vi "uService GUI.vi"(8 "error in (no error)":errorcluster, 11 "uService Template in":refnum<class "Scheduler.lvclass">=refnum) -> (3 "uService Template out":refnum<class "Scheduler.lvclass">)   [LabVIEW 2020, in "CIRCUS_uServices.lvlib" / "Scheduler.lvlib" / "Scheduler.lvclass"]
uses:
  Scheduler.lvclass
  Scheduler Consumer Case Selector.ctl
  Selection.ctl
  TALOS/TALOS_PPL.lvlibp/Father of all uServices/Father of all uServices/Father of all uServices.lvclass
  C:/Users/marco/Documents/GitHub_Lab/CIRCUS/TALOS/TALOS_PPL.lvlibp/Father of all uServices/Father of all uServices/Father of all uServices.lvclass
  C:/Users/marco/Documents/GitHub_Lab/CIRCUS/TALOS/TALOS_PPL.lvlibp/Ancestor/Ancestor/Ancestor.lvclass
  C:/Users/marco/Documents/GitHub_Lab/CIRCUS/TALOS/Actor Framework.lvlibp/1abvi3w/vi.lib/ActorFramework/Actor/Actor.lvclass
  Run Utilities/Sequence of SBlocks/Sequence of SBlcoks - GUI.ctl
  Run Utilities/Sequence of SBlocks/Sequence of SBlocks.lvclass
  Run Utilities/TypeDefs/Synchronize FPGA Cluster.ctl
  Run Utilities/Run Utilities.lvlib
  Run Utilities/Schedule Block/Schedule Block - simplified GUI.ctl
  Run Utilities/Schedule Block/Schedule Block.lvclass
panel:
  out "Sync. mask":T1[](array[typedef])
  in  "SB Buttons":T2
  in  "Reload parameters":bool
  in  "Append to":enum32{"Bottom", "Top"}(radio)
  in  "Parallel":bool
  in  "Array of Sequences":T3[](array[typedef])
  in  "Science":bool
  in  "Save":bool
  in  "Load":bool
  in  "Reset":bool
  in  "Add RUN":bool
  in  "stop Scheduler":bool
  # "SCHEDULER"
  # "Multi FPGA Operation"
  # "Sync. mask"
  # "Estimated time of execution"
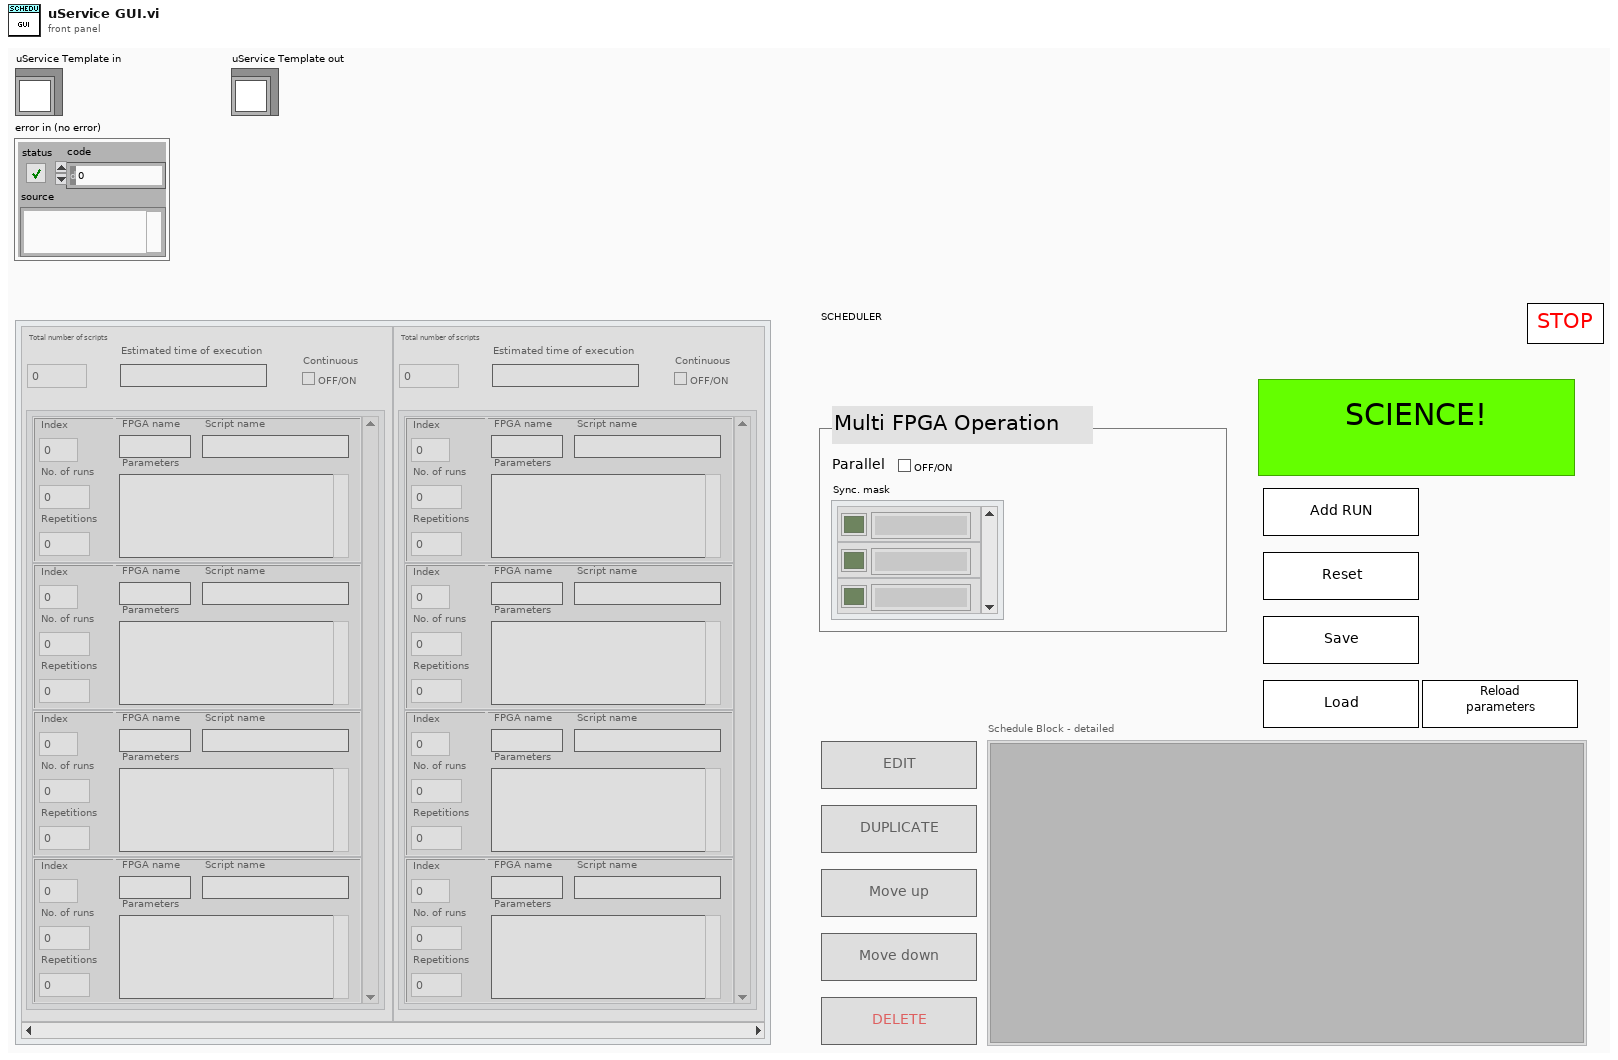
[diagram p1: front panel]
types:
  T1 = typedef "CIRCUS_uServices.lvlib/Run Utilities.lvlib/Synchronize FPGA Cluster.ctl" = cluster{"Status":bool, "FPGA Name":string}
  T2 = cluster{"Move up SB":bool, "Move down SB":bool, "DELETE_SB":bool, "DUPLICATE_SB":bool, "EDIT_SB":bool}
  T3 = typedef "CIRCUS_uServices.lvlib/Run Utilities.lvlib/Sequence of SBlocks.lvclass/Sequence of SBlcoks - GUI.ctl" = cluster{"Total number of scripts":i32, "Time":string, "Sequence of SBlocks":T4[], "Continuous":bool}
  T4 = typedef "CIRCUS_uServices.lvlib/Run Utilities.lvlib/Schedule Block.lvclass/Schedule Block - simplified GUI.ctl" = cluster{"Bcg Color":u32, "Index":i32, "No. of runs":i32, "Script name":string, "FPGA name":string, "Parameters":string, "Repetitions":i32}
  T5 = typedef "CIRCUS_uServices.lvlib/Scheduler.lvlib/Scheduler.lvclass/Scheduler Consumer Case Selector.ctl" = enum16{"Add SBlock", "Update GUI", "Move SBlock", "Select SBlock", "Update Cont.", "Load", "Save", "Reset", "Send to Tamer", "Edit SBlock", "Duplicate SBlock", "Delete SBlock", "Update SBlock", "Init", "Split/Combine Schedules", "Reschedule", "Load Parameters"}
  T6 = typedef "CIRCUS_uServices.lvlib/Scheduler.lvlib/Scheduler.lvclass/Selection.ctl" = cluster{"Row":i32, "Column":i32}
  T7 = typedef "TALOS.lvlib/Run Utilities.lvlib/Synchronize Kasli Cluster.ctl" = cluster{"Status":bool, "FPGA Name":string}
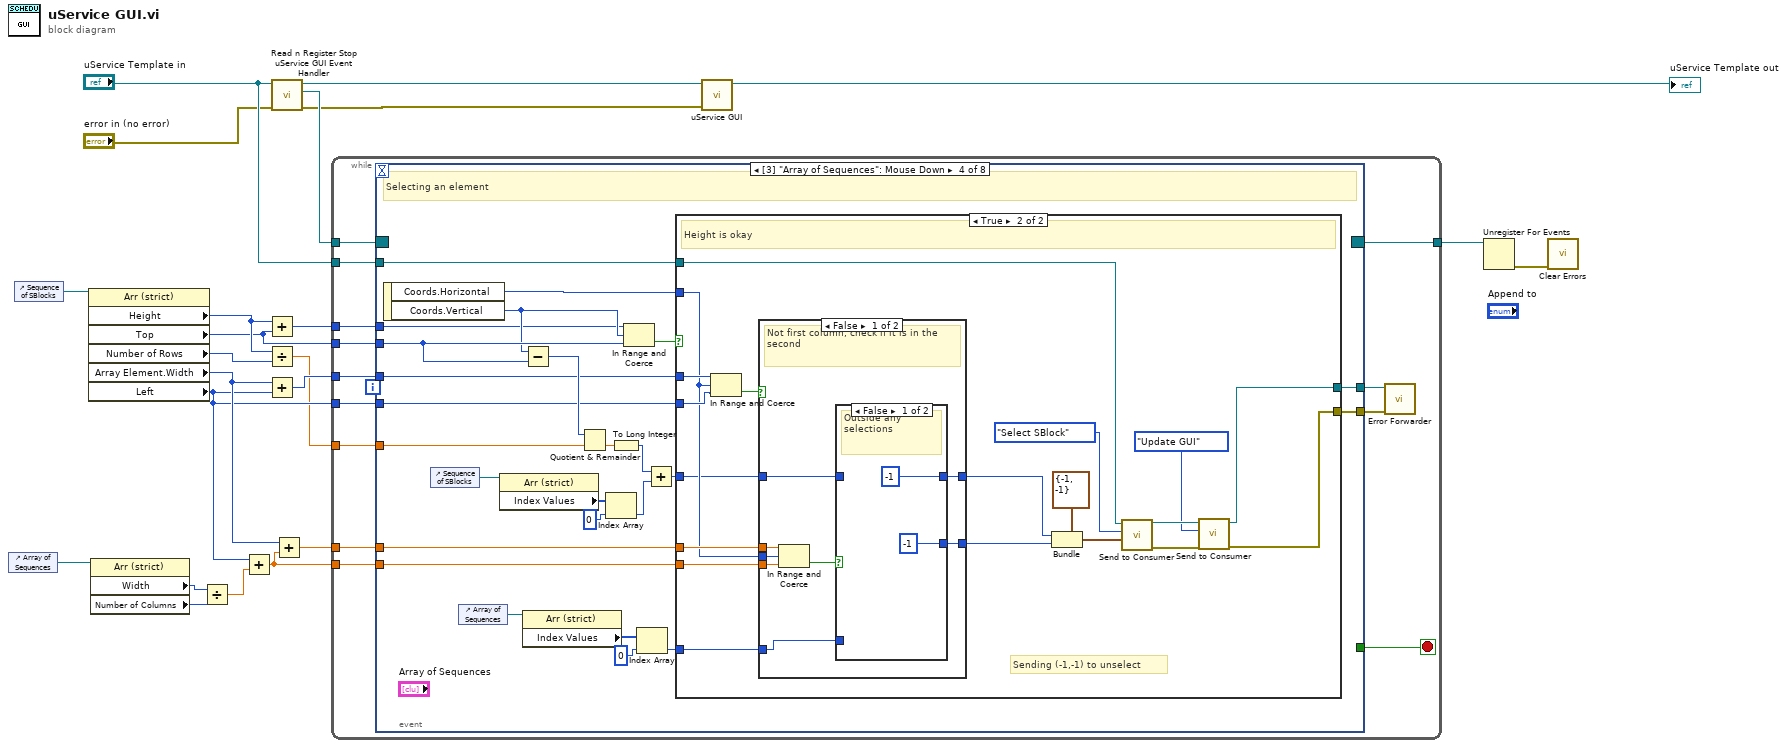
[diagram p0: block diagram]
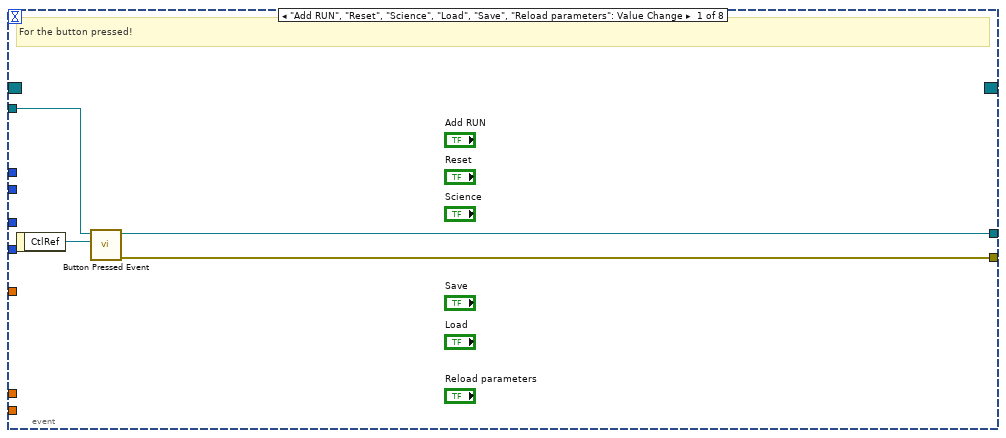
[diagram p2: hidden frame]
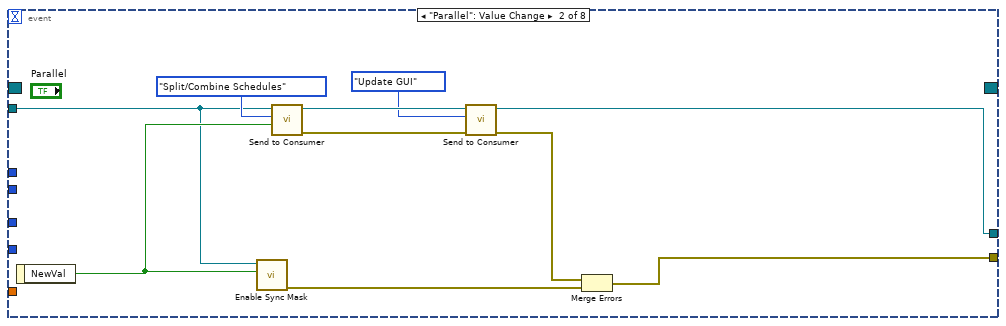
[diagram p3: hidden frame]
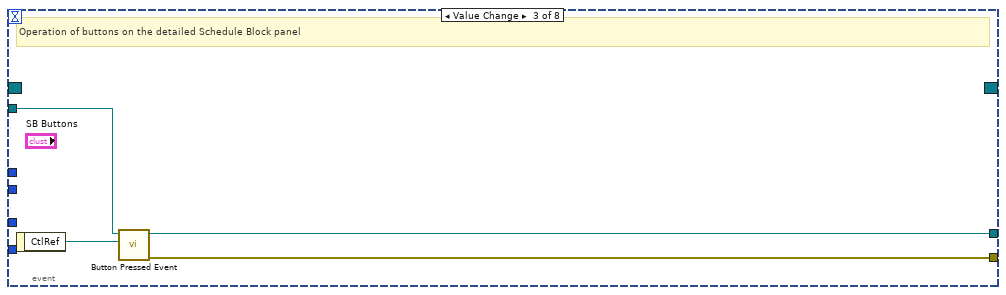
[diagram p4: hidden frame]
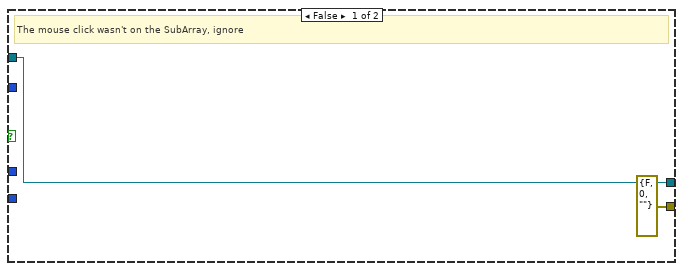
[diagram p5: hidden frame]
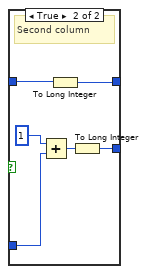
[diagram p6: hidden frame]
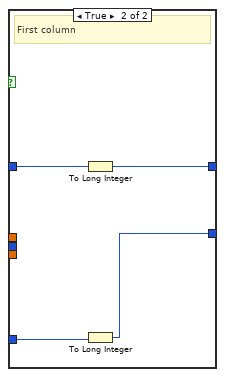
[diagram p7: hidden frame]
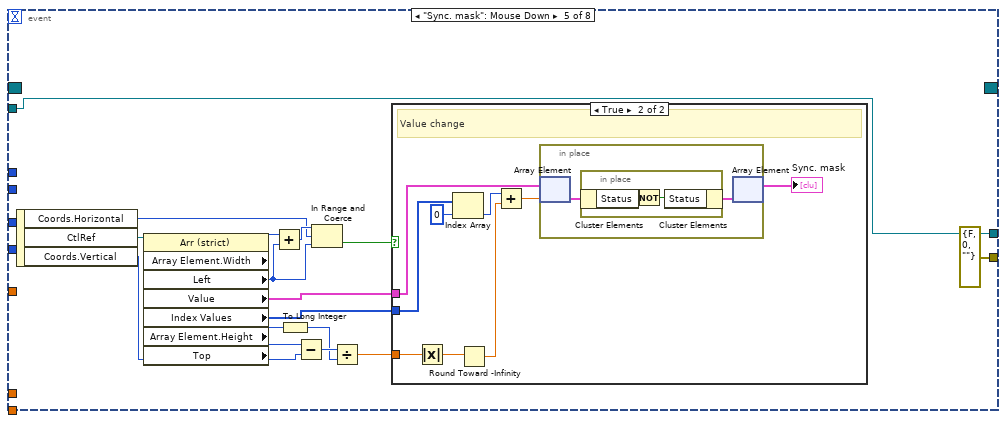
[diagram p8: hidden frame]
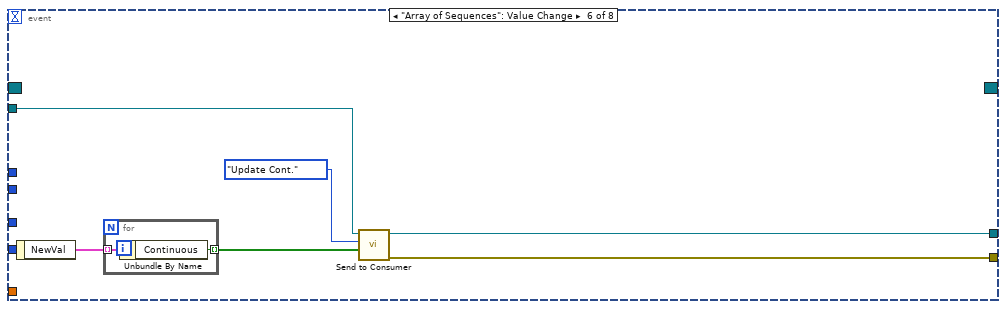
[diagram p10: hidden frame]
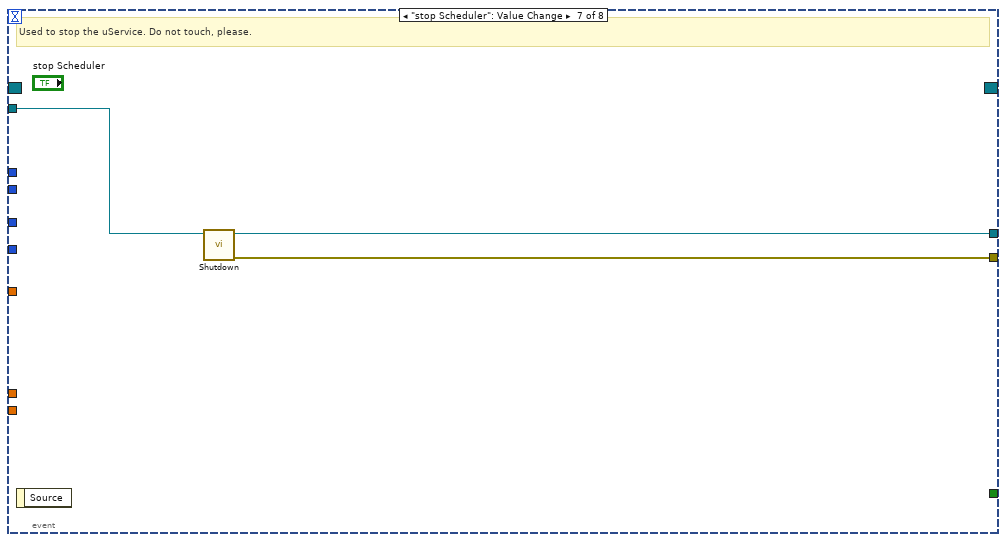
[diagram p11: hidden frame]
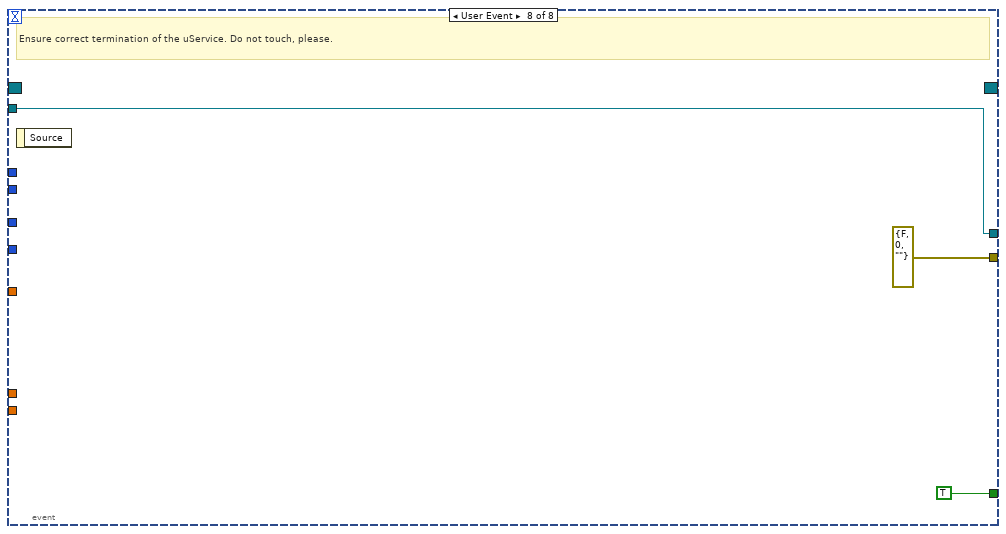
[diagram p12: hidden frame]
diagram:
  n1 = control-ref of="Array of Sequences"() -> (w5:refnum<vi>)
  n2 = control-ref of="Sequence of SBlocks"() -> (w4:refnum<vi>)
  n3 = property class="Arr (strict)"(reference=w4) -> ("Height"=w16:u32, "Top"=w11:i32, "Number of Rows"=w15:u32, "Array Element.Width"=w13:u32, "Left"=w9:i32)  [unwired: 1 in, 2 out]
  n4 = property class="Arr (strict)"(reference=w5) -> ("Width"=w17:u32, "Number of Columns"=w2:u32)  [unwired: 1 in, 2 out]
  n5 = Divide(x=w17, y=w2) -> (x/y=w14:dbl)
  n6 = Add(x=w9, y=w14) -> (x+y=w6:dbl)
  n7 = Add(x=w16, y=w11) -> (x+y=w12:u32)
  n8 = Divide(x=w16, y=w15) -> (x/y=w8:dbl)
  n9 = Add(x=w13, y=w9) -> (x+y=w10:u32)
  n10 = call-dynamic "Read n Register Stop uService GUI Event Handler .vi"("error in (no error)"="error in (no error)", "uService Template in"="uService Template in") -> ("error out"=w3:errorcluster, "Stop uService GUI Event Ref"=w18:refnum<event-registration>, "uService Template out"=w19:refnum<class "Scheduler.lvclass">)  [unwired: 7 in]
  n11 = Add(x=w13, y=w6) -> (x+y=w7:dbl)
  n12 = while {
    tunnel: [w36] -> w20
    tunnel: w18 -> [w34]
    tunnel: "uService Template in" -> [w33]
    tunnel: w12 -> [w32]
    tunnel: w11 -> [w31]
    tunnel: w10 -> [w30]
    tunnel: w9 -> [w29]
    tunnel: w8 -> [w28]
    tunnel: w7 -> [w27]
    tunnel: w6 -> [w26]
    stop <- w35 stop-if-true
    n13 = event shown="[3] \"Array of Sequences\": Mouse Down" {
      selector: w34 -> [_ _ _ _ _ _ _ _]
      dyn-events: [_ _ _ _ _ _ _ _] -> w36
      timeout: _ -> [_ _ _ _ _ _ _ _]
      tunnel: [_ _ _ _ _ _ _ TRUE] -> w35
      tunnel: w33 -> [w40 w45 w53 w61 w122 w154 w160 w162]
      tunnel: w32 -> [_ _ _ w57 _ _ _ _]
      tunnel: w31 -> [_ _ _ w68 _ _ _ _]
      tunnel: w30 -> [_ _ _ w67 _ _ _ _]
      tunnel: w29 -> [_ _ _ w66 _ _ _ _]
      tunnel: w28 -> [_ _ _ w65 _ _ _ _]
      tunnel: w27 -> [_ _ _ w64 _ _ _ _]
      tunnel: w26 -> [_ _ _ w58 _ _ _ _]
      tunnel: [w38 w41 w52 w56 w122 w151 w159 w162] -> w25
      tunnel: [w37 w42 w51 w55 errorcluster {"status"=FALSE, "code"=0, "source"=""} ("error out") w150 w158 errorcluster {"status"=FALSE, "code"=0, "source"=""} ("error out")] -> w24
      event "Add RUN", "Reset", "Science", "Load", "Save", "Reload parameters": Value Change {
        # "For the button pressed!"
        n14 = event-data() -> ("CtlRef"=w39:refnum<vi>)  [unwired: 1 in]
        n15 = call-dynamic "Button Pressed Event.vi"("CtlRef"=w39, "uService Template in"=w40) -> ("error out"=w37:errorcluster, "uService Template out"=w38:refnum<class "Scheduler.lvclass">)  [unwired: 8 in]
      }
      event "Parallel": Value Change {
        n16 = event-data() -> ("NewVal"=w46:bool)  [unwired: 1 in]
        n17 = call-dynamic "Enable Sync Mask.vi"("Enable"=w46, "Scheduler in"=w45) -> ("error out"=w43:errorcluster)  [unwired: 8 in, 1 out]
        n18 = call "Send to Consumer.vi"("Data"=w46, "Case ID"=Scheduler_Consumer_Case_Selector."Split/Combine Schedules" ("Shifter Panel Consumer Case Selector"), "uService Template in"=w45) -> ("error out"=w47:errorcluster, "uService Template out"=w50:refnum<class "Scheduler.lvclass">)  [unwired: 7 in]
        n19 = call "Send to Consumer.vi"("error in (no error)"=w47, "Case ID"=Scheduler_Consumer_Case_Selector."Update GUI" ("Shifter Panel Consumer Case Selector"), "uService Template in"=w50) -> ("error out"=w44:errorcluster, "uService Template out"=w41:refnum<class "Scheduler.lvclass">)  [unwired: 7 in]
        n20 = Merge Errors(w44, w43) -> (w42:errorcluster)
      }
      event "SB Buttons.Move up SB", "SB Buttons.Move down SB", "SB Buttons.DELETE_SB", "SB Buttons.DUPLICATE_SB", "SB Buttons.EDIT_SB": Value Change {
        # "Operation of buttons on the detailed Schedule Block panel"
        n21 = event-data() -> ("CtlRef"=w54:refnum<vi>)  [unwired: 1 in]
        n22 = call-dynamic "Button Pressed Event.vi"("CtlRef"=w54, "uService Template in"=w53) -> ("error out"=w51:errorcluster, "uService Template out"=w52:refnum<class "Scheduler.lvclass">)  [unwired: 8 in]
      }
      event "Array of Sequences": Mouse Down {
        # "Selecting an element"
        n23 = event-data() -> ("Coords.Horizontal"=w63:i32, "Coords.Vertical"=w62:i32)  [unwired: 1 in]
        n24 = control-ref of="Sequence of SBlocks"() -> (w60:refnum<vi>)
        n25 = control-ref of="Array of Sequences"() -> (w59:refnum<vi>)
        n26 = property class="Arr (strict)"(reference=w60) -> ("Index Values"=w73:u32[])  [unwired: 1 in, 2 out]
        n27 = Subtract(x=w62, y=w68) -> (x-y=w75:i32)
        n28 = property class="Arr (strict)"(reference=w59) -> ("Index Values"=w78:u32[])  [unwired: 1 in, 2 out]
        n29 = Quotient & Remainder(x=w75, y=w65) -> (floor(x/y)=w74:dbl)  [unwired: 1 out]
        n30 = Index Array(array=w73, index=0) -> (element=w70:u32)
        n31 = To Long Integer(number=w74) -> (32bit integer=w72:i32)
        n32 = In Range and Coerce(upper limit=w57, x=w62, lower limit=w68) -> (In Range?=w79:bool)  [unwired: 1 out]
        n33 = Index Array(array=w78, index=0) -> (element=w76:u32)
        n34 = Add(x=w72, y=w70) -> (x+y=w69:u32)
        n35 = case shown="True" w79 {
          tunnel: w67 -> [_ w100]
          tunnel: w66 -> [_ w99]
          tunnel: w63 -> [_ w95]
          tunnel: w64 -> [_ w97]
          tunnel: w58 -> [_ w96]
          tunnel: w76 -> [_ w94]
          tunnel: w69 -> [_ w93]
          tunnel: w61 -> [w81 w92]
          tunnel: [w81 w82] -> w56
          tunnel: [errorcluster {"status"=FALSE, "code"=0, "source"=""} ("error out") w83] -> w55
          frame False {
            # "The mouse click wasn't on the SubArray, ignore"
          }
          frame True {
            # "Sending (-1,-1) to unselect"
            # "Height is okay"
            n36 = In Range and Coerce(upper limit=w100, x=w95, lower limit=w99) -> (In Range?=w98:bool)  [unwired: 1 out]
            n37 = case shown="False" w98 {
              tunnel: w97 -> [w108 _]
              tunnel: w96 -> [w107 _]
              tunnel: w95 -> [w106 _]
              tunnel: w94 -> [w104 w118]
              tunnel: w93 -> [w103 w120]
              tunnel: [w102 w119] -> w91
              tunnel: [w101 w117] -> w90
              frame False {
                # "Not first column, check if it is in the second"
                n38 = In Range and Coerce(upper limit=w108, x=w106, lower limit=w107) -> (In Range?=w105:bool)  [unwired: 1 out]
                n39 = case shown="False" w105 {
                  tunnel: w104 -> [_ w115]
                  tunnel: w103 -> [_ w114]
                  tunnel: [-1 w113] -> w102
                  tunnel: [-1 w111] -> w101
                  frame False {
                    # "Outside any selections"
                  }
                  frame True {
                    # "Second column"
                    n40 = Add(x=1, y=w115) -> (x+y=w112:u32)
                    n41 = To Long Integer(number=w114) -> (32bit integer=w113:i32)
                    n42 = To Long Integer(number=w112) -> (32bit integer=w111:i32)
                  }
                }
              }
              frame True {
                # "First column"
                n43 = To Long Integer(number=w120) -> (32bit integer=w119:i32)
                n44 = To Long Integer(number=w118) -> (32bit integer=w117:i32)
              }
            }
            n45 = Bundle(cluster=T6 {"Row"=-1, "Column"=-1} ("Selection"), "Row"=w91, "Column"=w90) -> (w89:T6)
            n46 = call "Send to Consumer.vi"("Data"=w89, "Case ID"=Scheduler_Consumer_Case_Selector."Select SBlock" ("Shifter Panel Consumer Case Selector"), "uService Template in"=w92) -> ("error out"=w87:errorcluster, "uService Template out"=w85:refnum<class "Scheduler.lvclass">)  [unwired: 7 in]
            n47 = call "Send to Consumer.vi"("error in (no error)"=w87, "Case ID"=Scheduler_Consumer_Case_Selector."Update GUI" ("Shifter Panel Consumer Case Selector"), "uService Template in"=w85) -> ("error out"=w83:errorcluster, "uService Template out"=w82:refnum<class "Scheduler.lvclass">)  [unwired: 7 in]
          }
        }
      }
      event "Sync. mask": Mouse Down {
        n48 = event-data() -> ("Coords.Horizontal"=w132:i32, "CtlRef"=w136:refnum<vi>, "Coords.Vertical"=w126:i32)  [unwired: 1 in]
        n49 = property class="Arr (strict)"(reference=w136) -> ("Array Element.Width"=w134:u32, "Left"=w133:i32, "Value"=w129:T7[], "Index Values"=w128:u32[], "Array Element.Height"=w130:u32, "Top"=w127:i32)  [unwired: 1 in, 2 out]
        n50 = Add(x=w134, y=w133) -> (x+y=w135:u32)
        n51 = To Long Integer(number=w130) -> (32bit integer=w124:i32)
        n52 = Subtract(x=w127, y=w126) -> (x-y=w125:i32)
        n53 = In Range and Coerce(upper limit=w135, x=w132, lower limit=w133) -> (In Range?=w131:bool)  [unwired: 1 out]
        n54 = Divide(x=w125, y=w124) -> (x/y=w123:dbl)
        n55 = case shown="True" w131 {
          tunnel: w129 -> [_ w141]
          tunnel: w128 -> [_ w143]
          tunnel: w123 -> [_ w145]
          frame False {
            # "This is just scrolling"
          }
          frame True {
            # "Value change"
            n56 = Absolute Value(x=w145) -> (abs(x)=w144:dbl)
            n57 = Index Array(array=w143, index=0) -> (element=w139:u32)
            n58 = Round Toward -Infinity(1:w144) -> (0:w140:dbl)
            n59 = Add(x=w139, y=w140) -> (x+y=w138:dbl)
            n60 = in-place {
              n61 = in-place-array #1(w141, w138) -> (w147:T7)
              n62 = in-place {
                n63 = in-place-cluster #2(w147) -> ("Status"=w149:bool)
                n64 = Not(x=w149) -> (.not. x?=w148:bool)
                n65 = in-place-cluster #2("Status"=w148) -> (w146:T7)
              }
              n66 = in-place-array #1(w146) -> (→"Sync. mask":T7[])  [unwired: 1 out]
            }
          }
        }
      }
      event "Array of Sequences": Value Change {
        n67 = event-data() -> ("NewVal"=w155:T3[])  [unwired: 1 in]
        n68 = for {
          tunnel: w155 -> [w157] mode=indexing
          tunnel: [w156] -> w153 mode=indexing
          n69 = Unbundle By Name(w157) -> ("Continuous"=w156:bool)
        }
        n70 = call "Send to Consumer.vi"("Data"=w153, "Case ID"=Scheduler_Consumer_Case_Selector."Update Cont." ("Shifter Panel Consumer Case Selector"), "uService Template in"=w154) -> ("error out"=w150:errorcluster, "uService Template out"=w151:refnum<class "Scheduler.lvclass">)  [unwired: 7 in]
      }
      event "stop Scheduler": Value Change {
        # "Used to stop the uService. Do not touch, please."
        n71 = event-data() -> ()  [unwired: 1 in, 1 out]
        n72 = call "Shutdown.vi"("Father of all uServices in"=w160) -> ("error out"=w158:errorcluster, "Father of all uServices out"=w159:refnum<class "Scheduler.lvclass">)  [unwired: 9 in]
      }
      event User Event {
        # "Ensure correct termination of the uService. Do not touch, please."
        n73 = event-data() -> ()  [unwired: 1 in, 1 out]
      }
    }
    n74 = call "Error Forwarder.vi"("error in (no error)"=w24, "Father of all uServices in"=w25) -> ()  [unwired: 10 in]
  }
  n75 = call-parent "uService GUI.vi"("error in (no error)"=w3, "uService Template in"=w19) -> ("uService Template out"=→"uService Template out":refnum<class "Scheduler.lvclass">)  [unwired: 9 in]
  n76 = Unregister For Events(event registration refnum=w20) -> (error out=w1:errorcluster)  [unwired: 1 in]
  n77 = call <vilib>:"Clear Errors.vi"("error in (no error)"=w1) -> ()  [unwired: 5 in, 2 out]
